vi "calcupposfunc.vi"(8 "Step":i32, 9 "Pos":i32, 11 "Directon":string) -> (3 "Pos_Out":i32)   [LabVIEW 2011]
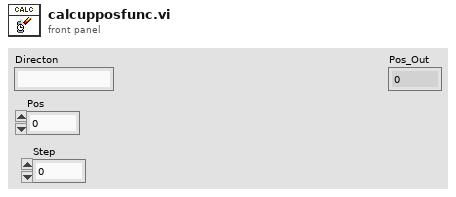
[diagram p1: front panel]
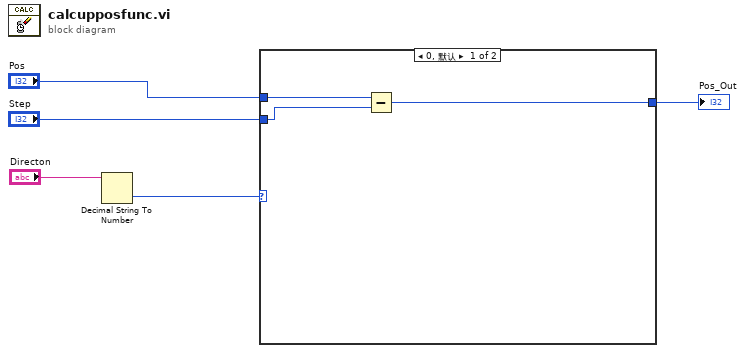
[diagram p0: block diagram]
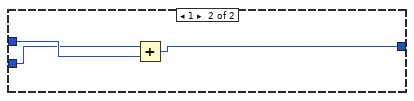
[diagram p2: hidden frame]
diagram:
  n1 = Decimal String To Number(string="Directon") -> (number=w4:i32)  [unwired: 2 in, 1 out]
  n2 = case shown="0, 默认" w4 {
    tunnel: "Pos" -> [w8 w11]
    tunnel: "Step" -> [w7 w10]
    tunnel: [w6 w9] -> w1
    frame 0, Default {
      n3 = Subtract(x=w8, y=w7) -> (x-y=w6:i32)
    }
    frame 1 {
      n4 = Add(x=w10, y=w11) -> (x+y=w9:i32)
    }
  }
  "Pos_Out" <- w1
